vi "ReadVarientData.vi"(11 "数组":variant[][](array[variant])) -> (0 "输出 6":dbl, 1 "输出 5":dbl, 2 "输出 3":dbl, 3 "输出 2":dbl, 4 "输出 4":dbl, 5 "输出 1":dbl)   [LabVIEW 2014]
uses:
  <vilib>/addons/database/_DB Variant To Data/Database Variant To Data.xnode
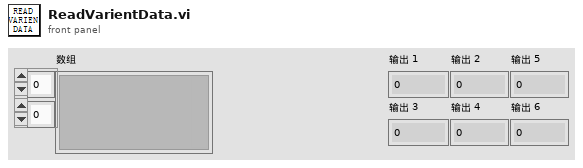
[diagram p1: front panel]
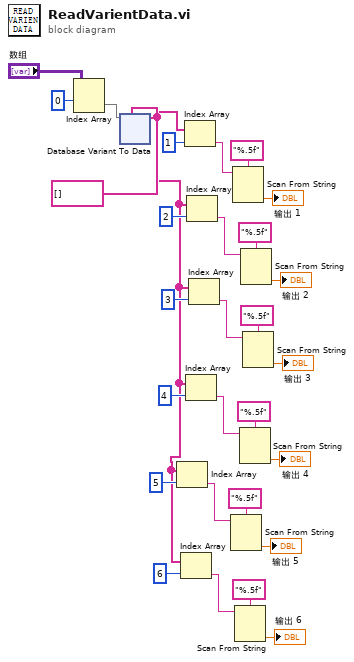
[diagram p0: block diagram]
diagram:
  n1 = Index Array(array="数组", index (row)=0 ("索引 (行)")) -> (element=w25:variant[])  [unwired: 1 in]
  n2 = xnode "Database Variant To Data"("database variant"=w25, "type"=string[] []) -> ("data"=w4:string[])  [unwired: 1 in, 1 out]
  n3 = Index Array(array=w4, index=5 ("索引")) -> (element=w9:string)
  n4 = Index Array(array=w4, index=6 ("索引")) -> (element=w8:string)
  n5 = Index Array(array=w4, index=1 ("索引")) -> (element=w22:string)
  n6 = Index Array(array=w4, index=4 ("索引")) -> (element=w14:string)
  n7 = Index Array(array=w4, index=2 ("索引")) -> (element=w29:string)
  n8 = Index Array(array=w4, index=3 ("索引")) -> (element=w15:string)
  n9 = Scan From String(format string="%.5f" ("格式字符串"), input string=w9) -> (output 1=→"输出 5":dbl)  [unwired: 3 in, 3 out]
  n10 = Scan From String(format string="%.5f" ("格式字符串"), input string=w22) -> (output 1=→"输出 1":dbl)  [unwired: 3 in, 3 out]
  n11 = Scan From String(format string="%.5f" ("格式字符串"), input string=w8) -> (output 1=→"输出 6":dbl)  [unwired: 3 in, 3 out]
  n12 = Scan From String(format string="%.5f" ("格式字符串"), input string=w14) -> (output 1=→"输出 4":dbl)  [unwired: 3 in, 3 out]
  n13 = Scan From String(format string="%.5f" ("格式字符串"), input string=w29) -> (output 1=→"输出 2":dbl)  [unwired: 3 in, 3 out]
  n14 = Scan From String(format string="%.5f" ("格式字符串"), input string=w15) -> (output 1=→"输出 3":dbl)  [unwired: 3 in, 3 out]
